vi "InfoResult.vi"(8 "error in":errorcluster, 11 "Result Step":T1) -> (0 "error out":errorcluster, 3 "Info Test":string)   [LabVIEW 2019]
doc: "Formatta le informazioni principali del risultato dell'update in una info box più leggibile"
uses:
  ByteGSAPIBase.lvclass
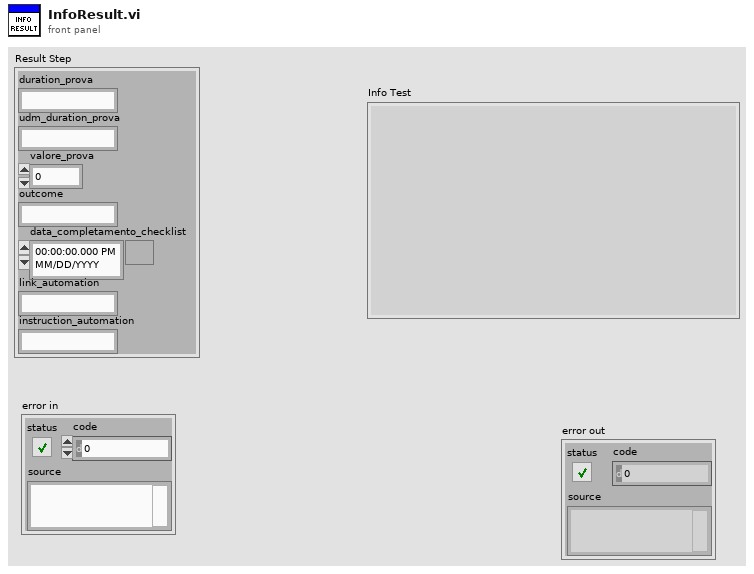
[diagram p1: front panel]
types:
  T1 = cluster{"duration_prova":string, "udm_duration_prova":string, "valore_prova":dbl, "outcome":string, "data_completamento_checklist":timestamp, "link_automation":string, "instruction_automation":string}
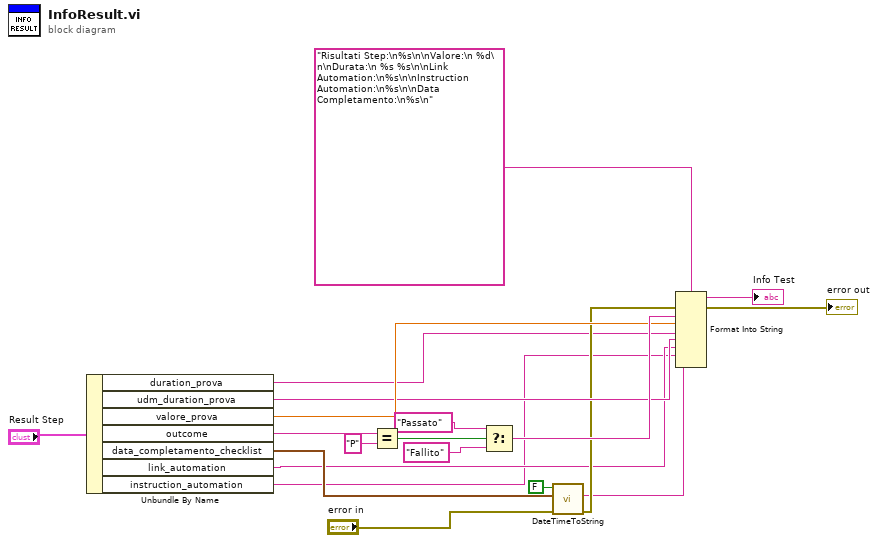
[diagram p0: block diagram]
diagram:
  n1 = Unbundle By Name("Result Step") -> ("duration_prova"=w5:string, "udm_duration_prova"=w10:string, "valore_prova"=w11:dbl, "outcome"=w20:string, "data_completamento_checklist"=w15:timestamp, "link_automation"=w3:string, "instruction_automation"=w2:string)
  n2 = Equal?(x=w20, y="P") -> (x = y?=w18:bool)
  n3 = Select(t="Passato" ("y"), s=w18, f="Fallito" ("y")) -> (s? t:f=w12:string)
  n4 = call "DateTimeToString.vi"("error in"="error in", "current time"=w15, "Time"=FALSE) -> ("error out"=w9:errorcluster, "Date string"=w1:string)  [unwired: 7 in]
  n5 = Format Into String(format string="Risultati Step:\n%s\n\nValore:\n %d\n\nDurata:\n %s %s\n\nLink Automation:\n%s\n\nInstruction Automation:\n%s\n\nData Completamento:\n%s\n", error in=w9, w12, w11, w5, w10, w3, w2, w1) -> (resulting string=→"Info Test":string, error out=→"error out":errorcluster)  [unwired: 1 in]
